vi "Configure Test.vi"(8 "error in (no error)":errorcluster) -> (0 "error out":errorcluster)   [LabVIEW 2015]
uses:
  Tests/Controls/Test Config.ctl
  Tests/Controls/Gas Mixture.ctl
  CAN Communication/PAS/Typedefs/ADC Gains.ctl
  Tests/Controls/Filter Sequence.ctl
  Tests/Controls/Functional Test.ctl
  CAN Communication/PAS/PAS.lvclass
panel:
  in  "Test Config":T1={"Chopper RPM"=140, "IR Power"=5, "Conc Tolerance"=0.0, "Gas Stable Time"=0, "A-D Settle"=0, "Samples"=0, "Filter Time"=0, "Gas Mixtures"=[], "Filter Sequences"=[], "Functional Test"={"Mic Test ON ADC Max"=0.0, "Mic Test ON ADC Min"=0.0, "Mic Test OFF ADC Max"=0.0, "Mic Test OFF ADC Min"=0.0, "Mic Test IC ADC Max"=0.0, "Mic Test IC ADC Min"=0.0, "IR Emitter ON ADC Max"=0.0, "IR Emitter ON ADC Min"=0.0, "IR Emitter OFF ADC Max"=0.0, "IR Emitter OFF ADC Min"=0.0}, "Initial Flow Rate"=0.0, "Max Flow Rate"=0.0} {"Gas Mixtures"."ADC Gains" items=["0"=0, "3"=3, "4"=4, "5"=5, "6"=6, "7"=7]; "Conc Tolerance" min=0.0 max=100.0 step=1.0; "IR Power" min=2 max=5 step=1; "Chopper RPM" min=140 max=1000 step=1}
  in  "Max Flow Rate":sgl caption="Max Flow Rate (ccm)"
  in  "Initial Flow Rate":sgl caption="Initial Flow Rate (ccm)"
  in  "Down Button":bool
  in  "Up Button":bool
  in  "Edit Gas":bool
  in  "Add Gas":bool
  in  "Remove Gas":bool
  in  "Gas Stable Time":u16 caption="Gas Stability Time (s)"
  in  "Conc Tolerance":dbl caption="Concentration Tolerance (%)" min=0.0 max=100.0 step=1.0
  in  "Gas Mixtures":i32(listbox)=-2
  out "Cancelled?":bool
  in  "Cancel Button":bool
  in  "OK Button":bool
  out "Test Sequence":i32(listbox)=-2
  # "Configure Test"
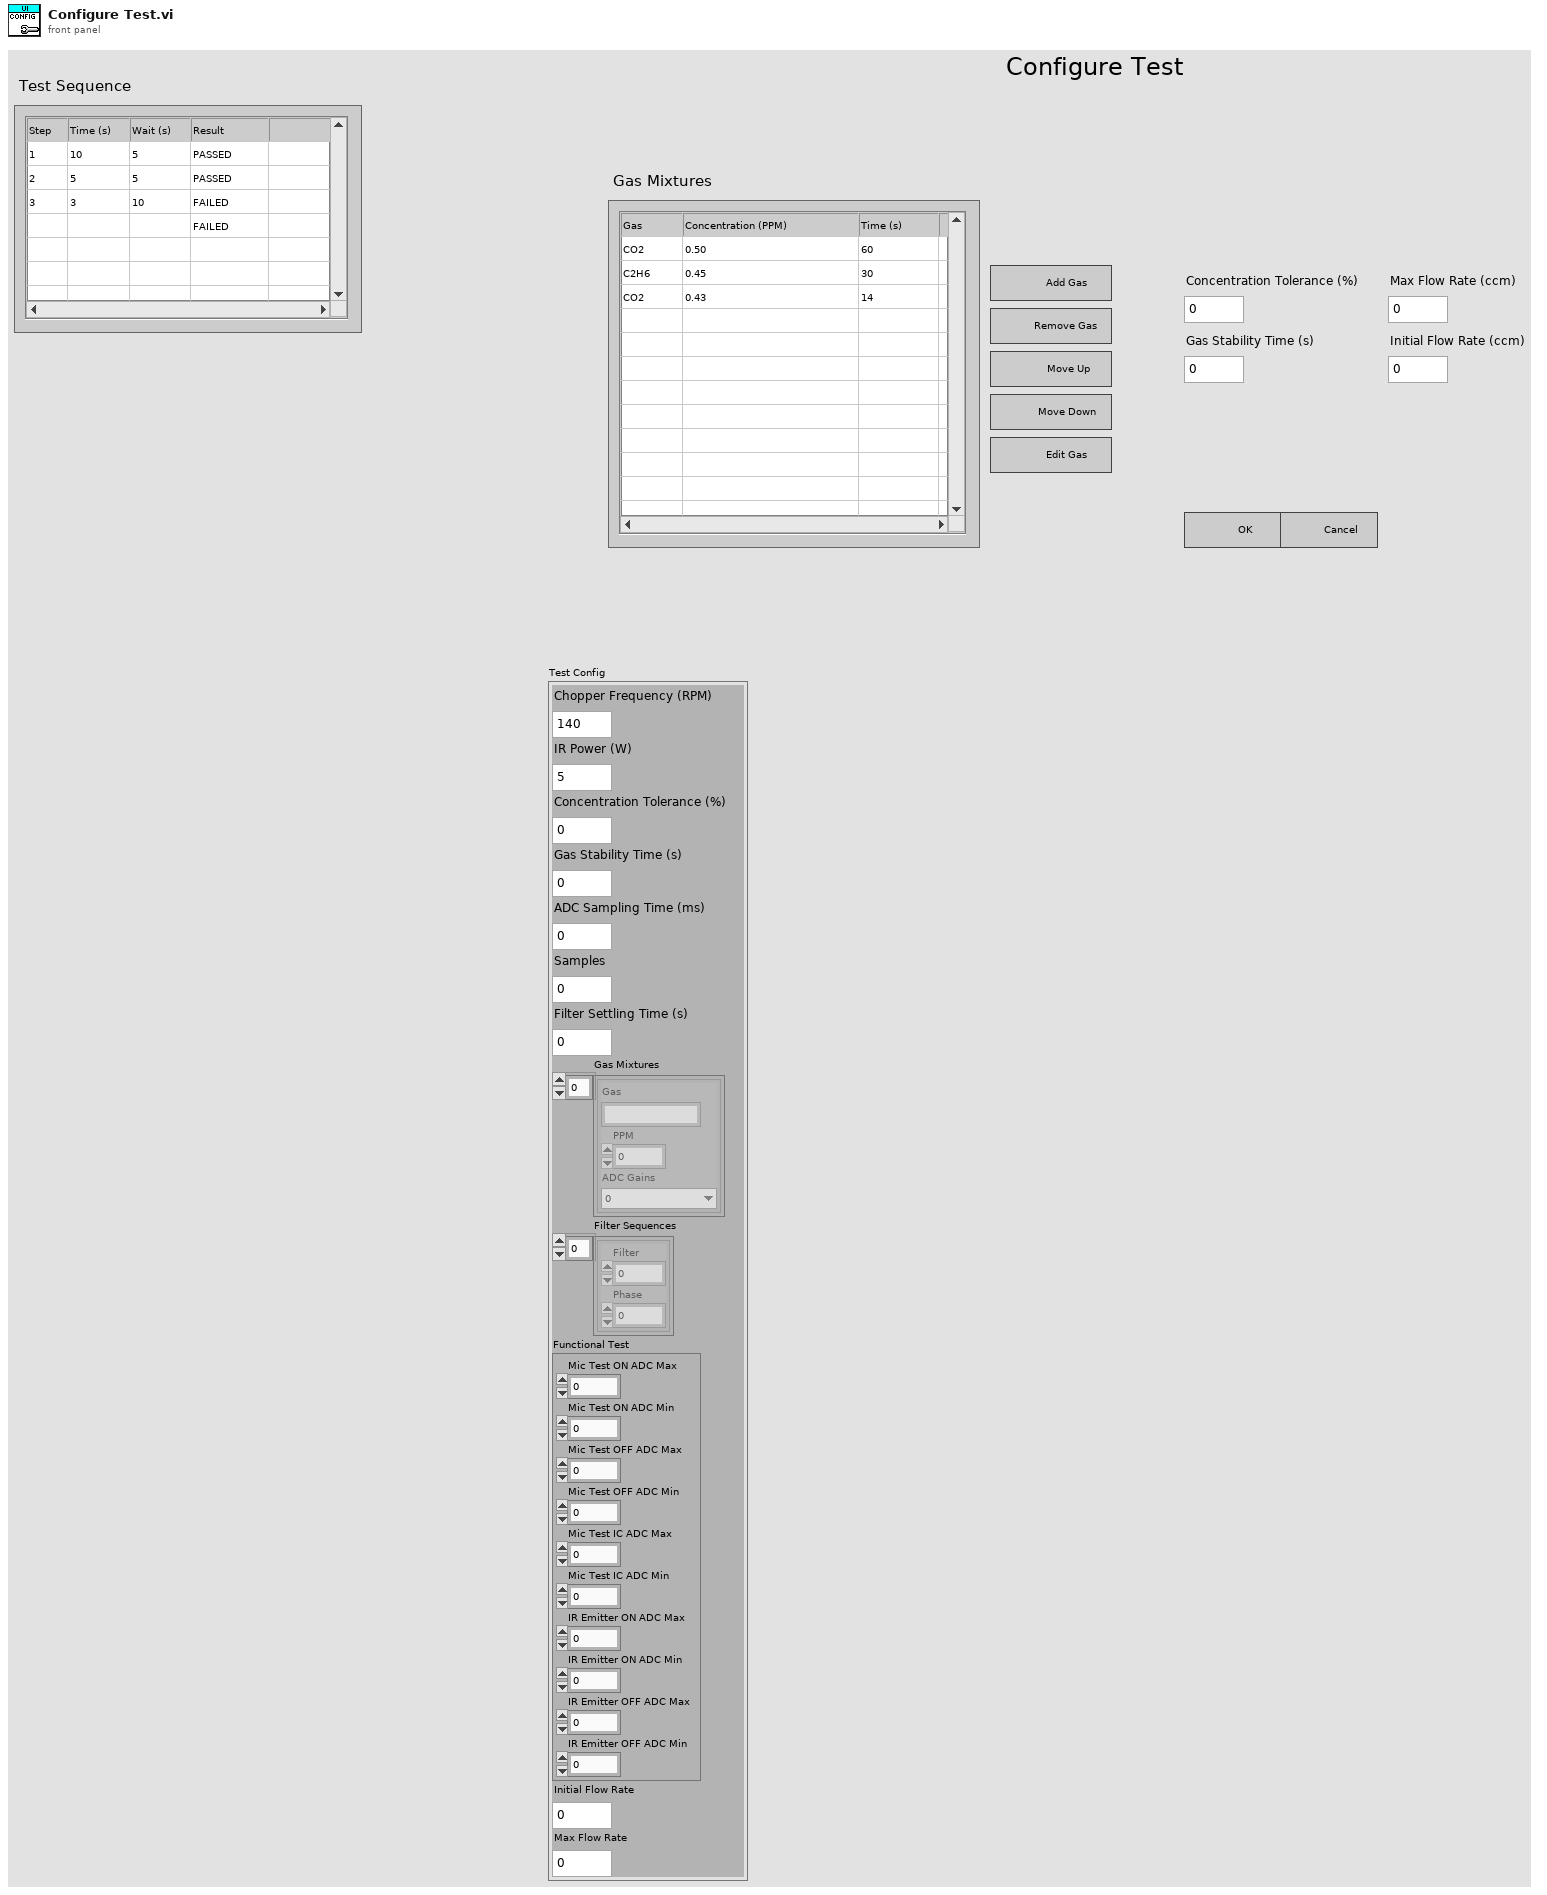
[diagram p1: front panel]
types:
  T1 = typedef "Test Config.ctl" = cluster{"Chopper RPM":u16, "IR Power":u8, "Conc Tolerance":dbl, "Gas Stable Time":u16, "A-D Settle":u16, "Samples":u16, "Filter Time":u16, "Gas Mixtures":T2[], "Filter Sequences":T4[], "Functional Test":T5, "Initial Flow Rate":sgl, "Max Flow Rate":sgl}
  T2 = typedef "Gas Mixture.ctl" = cluster{"Gas":string, "PPM":dbl, "ADC Gains":T3}
  T3 = typedef "PAS.lvclass/ADC Gains.ctl" = u16
  T4 = typedef "Filter Sequence.ctl" = cluster{"Filter":u8, "Phase":dbl}
  T5 = typedef "Functional Test.ctl" = cluster{"Mic Test ON ADC Max":dbl, "Mic Test ON ADC Min":dbl, "Mic Test OFF ADC Max":dbl, "Mic Test OFF ADC Min":dbl, "Mic Test IC ADC Max":dbl, "Mic Test IC ADC Min":dbl, "IR Emitter ON ADC Max":dbl, "IR Emitter ON ADC Min":dbl, "IR Emitter OFF ADC Max":dbl, "IR Emitter OFF ADC Min":dbl}
  T6 = typedef "Master Config.ctl" = cluster{"Conc Tolerance":dbl, "Gas Stable Time":u16, "Initial Flow Rate":sgl, "Max Flow Rate":sgl, "Gas Sequence":T7[]}
  T7 = typedef "Gas Info.ctl" = cluster{"Gas":string, "PPM":dbl, "Time":u32}
  T8 = typedef "LVPoint32TypeDef.ctl" = cluster{"Horizontal":i32, "Vertical":i32}
  T9 = typedef "LVRowAndColumnTypeDef.ctl" = cluster{"Row":i32, "Column":i32}
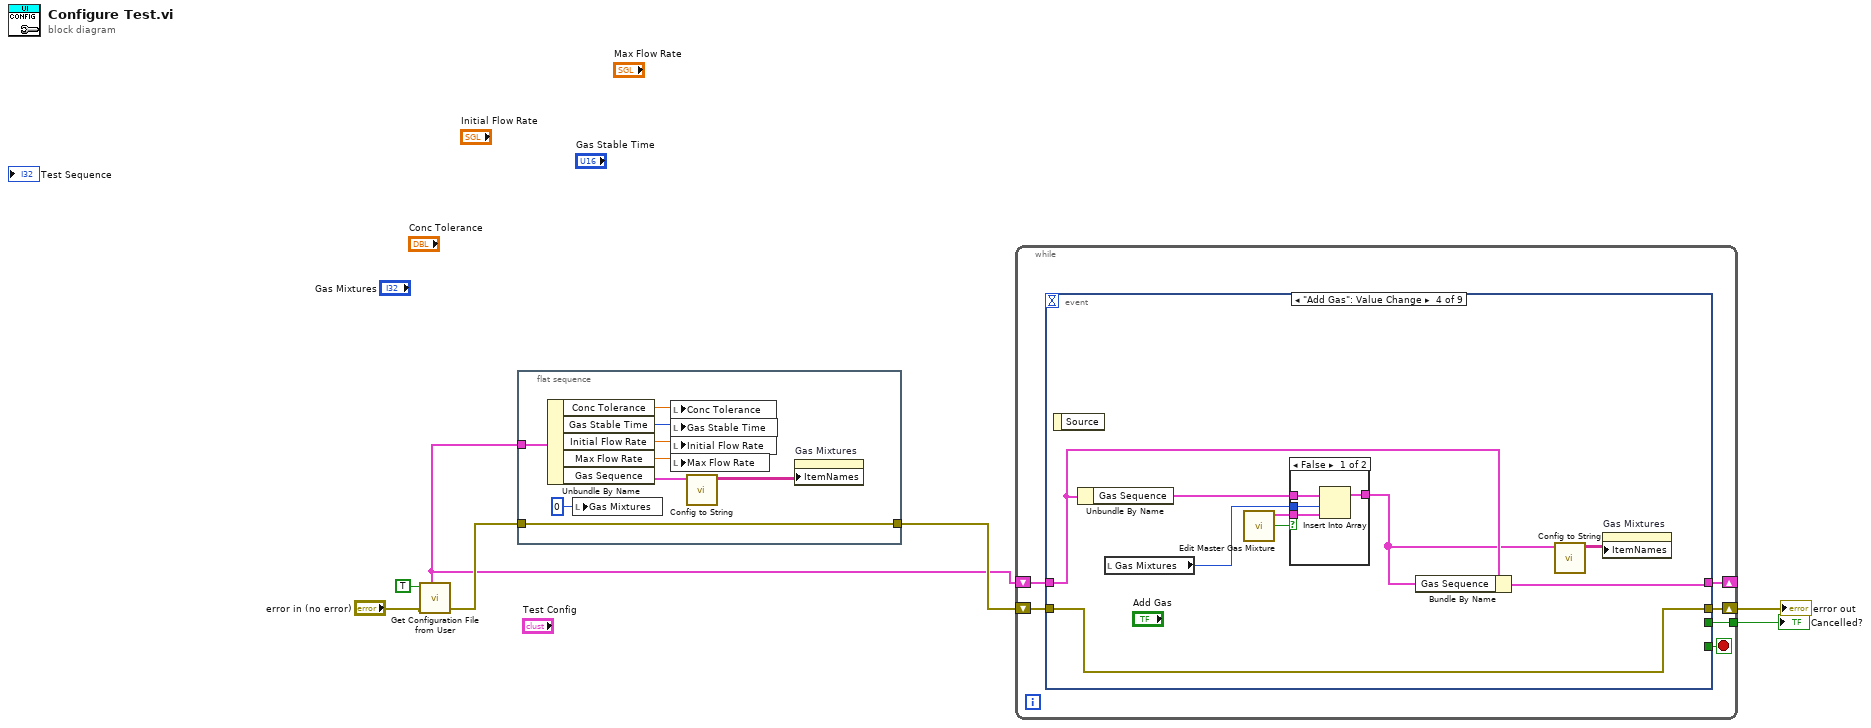
[diagram p0: block diagram]
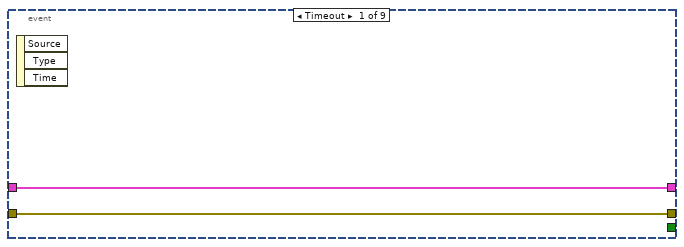
[diagram p2: hidden frame]
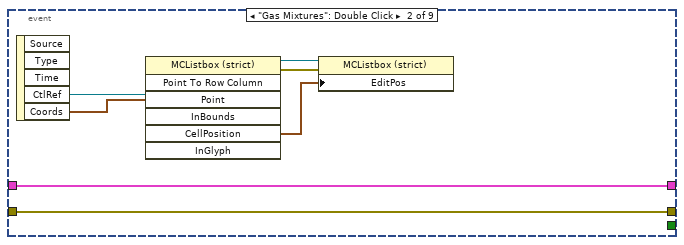
[diagram p3: hidden frame]
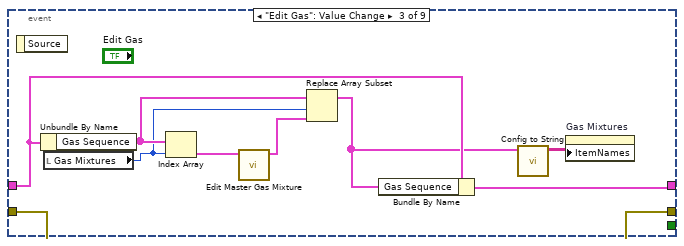
[diagram p4: hidden frame]
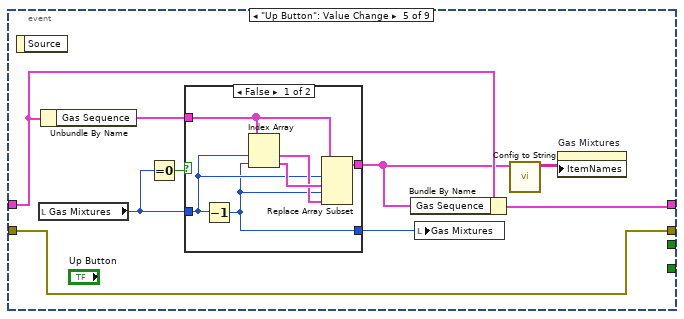
[diagram p6: hidden frame]
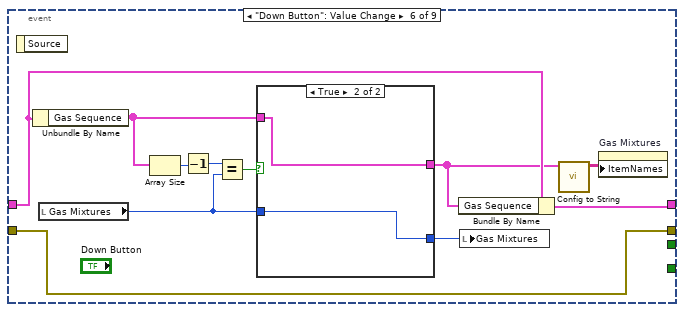
[diagram p8: hidden frame]
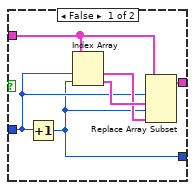
[diagram p9: hidden frame]
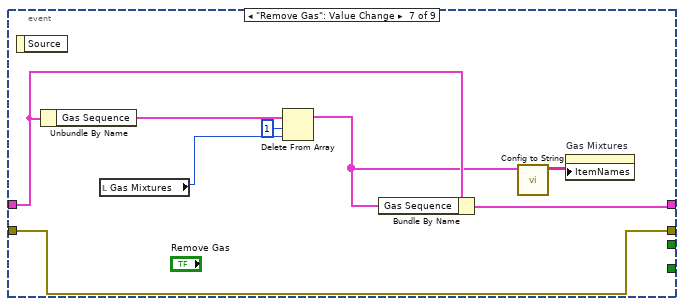
[diagram p10: hidden frame]
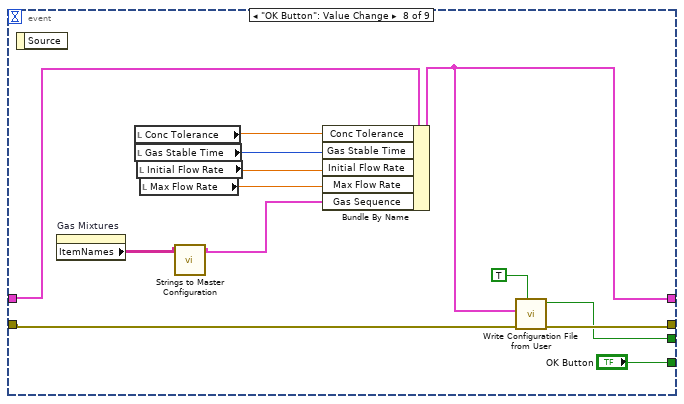
[diagram p11: hidden frame]
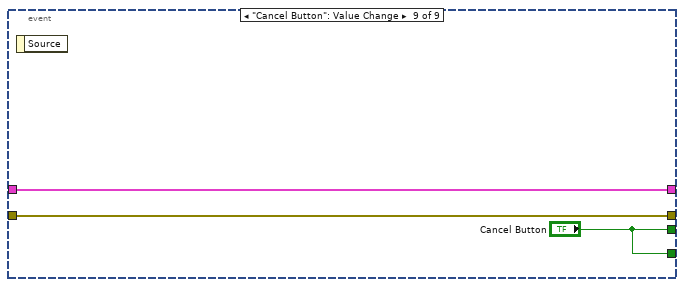
[diagram p12: hidden frame]
diagram:
  n1 = call "Get Configuration File from User.vi"("error in"="error in (no error)", "Master?"=TRUE) -> ("error out"=w3:errorcluster, "Master Config"=w2:T6)  [unwired: 6 in, 2 out]
  n2 = flat-sequence {
    tunnel: w2 -> [w15]
    tunnel: w3 -> [w16]
    tunnel: [w16] -> w5
    frame #0 {
      n3 = Unbundle By Name(w15) -> ("Conc Tolerance"=w14:dbl, "Gas Stable Time"=w13:u16, "Initial Flow Rate"=w11:sgl, "Max Flow Rate"=w10:sgl, "Gas Sequence"=w9:T7[])
      n4 = local write "Gas Mixtures"(0 ("Gas Mixtures")) -> ()
      n5 = local write "Conc Tolerance"(w14) -> ()
      n6 = local write "Gas Stable Time"(w13) -> ()
      n7 = local write "Initial Flow Rate"(w11) -> ()
      n8 = local write "Max Flow Rate"(w10) -> ()
      n9 = call "Config to String.vi"("Gas Sequence"=w9) -> ("Gas"=w12:string[][])  [unwired: 10 in]
      n10 = property on="Gas Mixtures" class="MCListbox (strict)"("ItemNames"=w12) -> ()  [unwired: 2 in, 2 out]
    }
  }
  n11 = while {
    tunnel: [w22] -> w7
    shift-right: [w19] -> w6
    shift-left: w5 -> [w20]
    shift-right: [w17] -> _
    shift-left: w2 -> [w18]
    stop <- w21 stop-if-true
    n12 = event shown="[3] \"Add Gas\": Value Change" {
      selector: _ -> [_ _ _ _ _ _ _ _ _]
      dyn-events: _ -> [_ _ _ _ _ _ _ _ _]
      timeout: _ -> [_ _ _ _ _ _ _ _ _]
      tunnel: [_ _ _ _ _ _ _ w107 "Cancel Button"] -> w22
      tunnel: [_ _ _ _ _ _ _ "OK Button" "Cancel Button"] -> w21
      tunnel: w20 -> [w24 w26 w39 w49 w63 w82 w98 w109 w113]
      tunnel: [w24 w26 w39 w49 w63 w82 w98 w110 w113] -> w19
      tunnel: w18 -> [w23 w25 w35 w47 w62 w81 w97 w108 w112]
      tunnel: [w23 w25 w34 w46 w61 w80 w96 w99 w112] -> w17
      event Timeout {
        n13 = event-data() -> ()  [unwired: 1 in, 3 out]
      }
      event "Gas Mixtures": Double Click {
        n14 = event-data() -> ("CtlRef"=w31:refnum<vi>, "Coords"=w30:T8)  [unwired: 1 in, 3 out]
        n15 = invoke class="MCListbox (strict)" method="Point To Row Column"(reference=w31, "Point"=w30) -> (reference out=w29:refnum<vi>, error out=w28:errorcluster, "CellPosition"=w27:T9)  [unwired: 5 in, 4 out]
        n16 = property class="MCListbox (strict)"(reference=w29, error in=w28, "EditPos"=w27) -> ()  [unwired: 2 out]
      }
      event "Edit Gas": Value Change {
        n17 = event-data() -> ()  [unwired: 1 in, 1 out]
        n18 = Unbundle By Name(w35) -> ("Gas Sequence"=w38:T7[])
        n19 = local read "Gas Mixtures"() -> (w37:i32)
        n20 = Index Array(array=w38, index=w37) -> (element=w40:T7)
        n21 = call "Edit Master Gas Mixture.vi"("Gas Info"=w40) -> ("Gas Info Out"=w36:T7)  [unwired: 8 in, 2 out]
        n22 = Replace Array Subset(array=w38, new element=w36, index=w37) -> (w33:T7[])
        n23 = Bundle By Name(cluster=w35, "Gas Sequence"=w33) -> (w34:T6)
        n24 = call "Config to String.vi"("Gas Sequence"=w33) -> ("Gas"=w32:string[][])  [unwired: 10 in]
        n25 = property on="Gas Mixtures" class="MCListbox (strict)"("ItemNames"=w32) -> ()  [unwired: 2 in, 2 out]
      }
      event "Add Gas": Value Change {
        n26 = event-data() -> ()  [unwired: 1 in, 1 out]
        n27 = Unbundle By Name(w47) -> ("Gas Sequence"=w43:T7[])
        n28 = local read "Gas Mixtures"() -> (w41:i32)
        n29 = call "Edit Master Gas Mixture.vi"() -> ("Cancel?"=w42:bool, "Gas Info Out"=w48:T7)  [unwired: 9 in, 1 out]
        n30 = case shown="False" w42 {
          tunnel: w41 -> [w53 _]
          tunnel: w48 -> [w52 _]
          tunnel: [w51 w54] -> w45
          tunnel: w43 -> [w50 w54]
          frame False {
            n31 = Insert Into Array(array=w50, index=w53, new element=w52) -> (w51:T7[])
          }
          frame True {
          }
        }
        n32 = Bundle By Name(cluster=w47, "Gas Sequence"=w45) -> (w46:T6)
        n33 = call "Config to String.vi"("Gas Sequence"=w45) -> ("Gas"=w44:string[][])  [unwired: 10 in]
        n34 = property on="Gas Mixtures" class="MCListbox (strict)"("ItemNames"=w44) -> ()  [unwired: 2 in, 2 out]
      }
      event "Up Button": Value Change {
        n35 = event-data() -> ()  [unwired: 1 in, 1 out]
        n36 = local read "Gas Mixtures"() -> (w57:i32)
        n37 = Unbundle By Name(w62) -> ("Gas Sequence"=w59:T7[])
        n38 = Equal To 0?(x=w57) -> (x = 0?=w56:bool)
        n39 = case shown="False" w56 {
          tunnel: w59 -> [w69 w71]
          tunnel: [w66 w71] -> w58
          tunnel: w57 -> [w65 w70]
          tunnel: [w64 w70] -> w55
          frame False {
            n40 = Decrement(x=w65) -> (x-1=w64:i32)
            n41 = Index Array(array=w69, index #1=w65, index #2=w64) -> (element #1=w67:T7, element #2=w68:T7)
            n42 = Replace Array Subset(array=w69, new element #1=w68, index #1=w65, new element #2=w67, index #2=w64) -> (w66:T7[])
          }
          frame True {
          }
        }
        n43 = Bundle By Name(cluster=w62, "Gas Sequence"=w58) -> (w61:T6)
        n44 = local write "Gas Mixtures"(w55) -> ()
        n45 = call "Config to String.vi"("Gas Sequence"=w58) -> ("Gas"=w60:string[][])  [unwired: 10 in]
        n46 = property on="Gas Mixtures" class="MCListbox (strict)"("ItemNames"=w60) -> ()  [unwired: 2 in, 2 out]
      }
      event "Down Button": Value Change {
        n47 = event-data() -> ()  [unwired: 1 in, 1 out]
        n48 = Unbundle By Name(w81) -> ("Gas Sequence"=w77:T7[])
        n49 = local read "Gas Mixtures"() -> (w74:i32)
        n50 = Array Size(array=w77) -> (size(s)=w76:i32)
        n51 = Decrement(x=w76) -> (x-1=w75:i32)
        n52 = Equal?(x=w75, y=w74) -> (x = y?=w73:bool)
        n53 = case shown="True" w73 {
          tunnel: w77 -> [w88 w90]
          tunnel: [w85 w90] -> w78
          tunnel: w74 -> [w84 w89]
          tunnel: [w83 w89] -> w72
          frame False {
            n54 = Increment(x=w84) -> (x+1=w83:i32)
            n55 = Index Array(array=w88, index #1=w84, index #2=w83) -> (element #1=w86:T7, element #2=w87:T7)
            n56 = Replace Array Subset(array=w88, new element #1=w87, index #1=w84, new element #2=w86, index #2=w83) -> (w85:T7[])
          }
          frame True {
          }
        }
        n57 = Bundle By Name(cluster=w81, "Gas Sequence"=w78) -> (w80:T6)
        n58 = local write "Gas Mixtures"(w72) -> ()
        n59 = call "Config to String.vi"("Gas Sequence"=w78) -> ("Gas"=w79:string[][])  [unwired: 10 in]
        n60 = property on="Gas Mixtures" class="MCListbox (strict)"("ItemNames"=w79) -> ()  [unwired: 2 in, 2 out]
      }
      event "Remove Gas": Value Change {
        n61 = event-data() -> ()  [unwired: 1 in, 1 out]
        n62 = Unbundle By Name(w97) -> ("Gas Sequence"=w93:T7[])
        n63 = local read "Gas Mixtures"() -> (w92:i32)
        n64 = Delete From Array(array=w93, length=1, index=w92) -> (array with subset deleted=w95:T7[])  [unwired: 1 out]
        n65 = Bundle By Name(cluster=w97, "Gas Sequence"=w95) -> (w96:T6)
        n66 = call "Config to String.vi"("Gas Sequence"=w95) -> ("Gas"=w94:string[][])  [unwired: 10 in]
        n67 = property on="Gas Mixtures" class="MCListbox (strict)"("ItemNames"=w94) -> ()  [unwired: 2 in, 2 out]
      }
      event "OK Button": Value Change {
        n68 = event-data() -> ()  [unwired: 1 in, 1 out]
        n69 = property on="Gas Mixtures" class="MCListbox (strict)"() -> ("ItemNames"=w102:string[][])  [unwired: 2 in, 2 out]
        n70 = local read "Conc Tolerance"() -> (w106:dbl)
        n71 = local read "Gas Stable Time"() -> (w105:u16)
        n72 = local read "Initial Flow Rate"() -> (w104:sgl)
        n73 = local read "Max Flow Rate"() -> (w103:sgl)
        n74 = call "Strings to Master Configuration.vi"("Gas"=w102) -> ("Gas Sequence"=w101:T7[])  [unwired: 10 in]
        n75 = Bundle By Name(cluster=w108, "Conc Tolerance"=w106, "Gas Stable Time"=w105, "Initial Flow Rate"=w104, "Max Flow Rate"=w103, "Gas Sequence"=w101) -> (w99:T6)
        n76 = call "Write Configuration File from User.vi"("Master?"=TRUE, "error in"=w109, "Master Config"=w99) -> ("error out"=w110:errorcluster, "Cancelled?"=w107:bool)  [unwired: 7 in]
      }
      event "Cancel Button": Value Change {
        n77 = event-data() -> ()  [unwired: 1 in, 1 out]
      }
    }
  }
  "error out" <- w6
  "Cancelled?" <- w7
